vi "Samples Needed.vi"(9 "Threshold":dbl, 11 "Sample Array":dbl[](array[numeric])) -> (1 "Index":dbl, 3 "Samples Needed":i32)   [LabVIEW 2012]
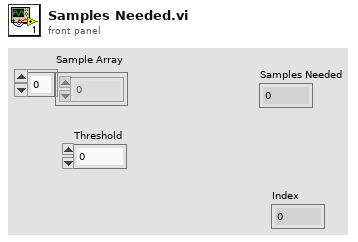
[diagram p1: front panel]
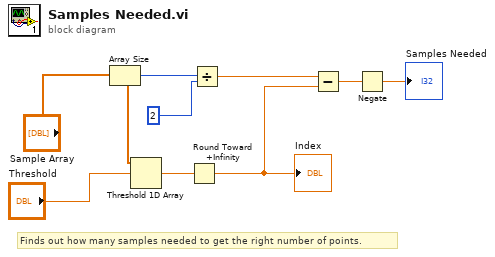
[diagram p0: block diagram]
diagram:
  # "Finds out how many samples needed to get the right number of points."
  n1 = Array Size(array="Sample Array") -> (size(s)=w6:i32)
  n2 = Threshold 1D Array(2:"Threshold", 3:"Sample Array") -> (0:w9:dbl)  [unwired: 1 in]
  n3 = Round Toward +Infinity(x=w9) -> (ceil(x): smallest int >= x=w1:dbl)
  "Index" <- w1
  n4 = Divide(x=w6, y=2) -> (x/y=w4:dbl)
  n5 = Subtract(x=w4, y=w1) -> (x-y=w3:dbl)
  n6 = Negate(x=w3) -> (-x=→"Samples Needed":dbl)
